vi "MoveOneStep.vi"(8 "error in (no error)":errorcluster, 11 "2D_Representer in":refnum<class "2D_Representer.lvclass">) -> (0 "error out":errorcluster, 3 "2D_Representer out":refnum<class "2D_Representer.lvclass">)   [LabVIEW 2018, in "2D_Representer.lvclass"]
uses:
  2D_Representer.lvclass
  2D_Representer.lvclass/2D_Representer.ctl
  Snake/Snake.lvclass
  Feeder/Feeder.lvclass
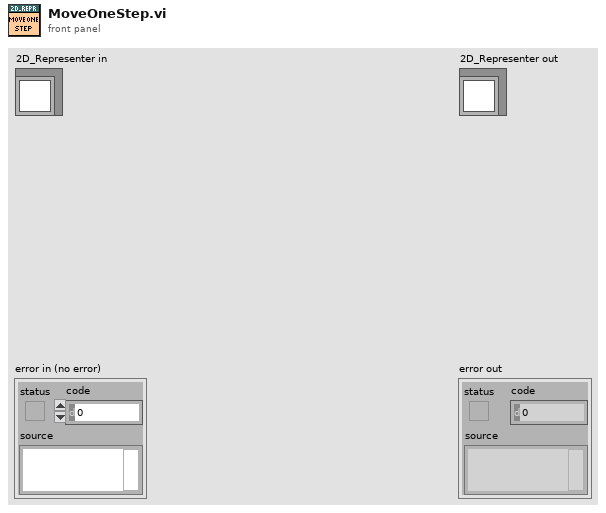
[diagram p1: front panel]
types:
  T1 = typedef "XYposition.ctl" = cluster{"Col.LocX":i32, "Row.LocY":i32}
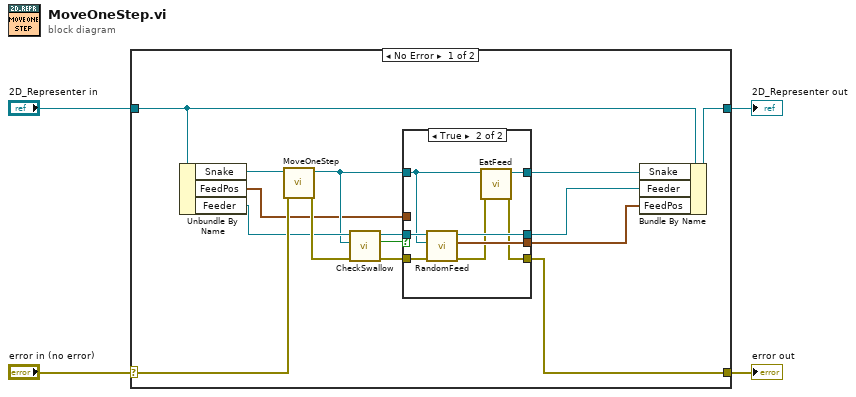
[diagram p0: block diagram]
diagram:
  n1 = case shown="No Error" "error in (no error)" {
    selector: "error in (no error)" -> [w16 w33]
    tunnel: [w12 w33] -> w3
    tunnel: [w17 w32] -> w1
    tunnel: "2D_Representer in" -> [w19 w32]
    frame No Error {
      n2 = Unbundle By Name(w19) -> ("Snake"=w18:refnum<class "Snake.lvclass">, "FeedPos"=w6:T1, "Feeder"=w13:refnum<class "Feeder.lvclass">)
      n3 = call "MoveOneStep.vi"("error in (no error)"=w16, "Snake in"=w18) -> ("error out"=w15:errorcluster, "Snake out"=w9:refnum<class "Snake.lvclass">)  [unwired: 8 in]
      n4 = call "CheckSwallow.vi"("error in (no error)"=w15, "Snake.lvclass"=w9, "Feeder in"=w13) -> ("error out"=w14:errorcluster, "Swallowed?"=w11:bool, "Feeder out"=w10:refnum<class "Feeder.lvclass">)  [unwired: 6 in]
      n5 = case shown="True" w11 {
        tunnel: w14 -> [w23 w31]
        tunnel: [w23 w24] -> w12
        tunnel: w10 -> [w22 w30]
        tunnel: w9 -> [w20 w27]
        tunnel: [w22 w29] -> w8
        tunnel: [w21 w28] -> w7
        tunnel: w6 -> [w21 _]
        tunnel: [w20 w26] -> w5
        frame False {
        }
        frame True {
          n6 = call "RandomFeed.vi"("error in (no error)"=w31, "Snake"=w27, "Feeder in"=w30) -> ("error out"=w25:errorcluster, "FeedPos"=w28:T1, "Feeder out"=w29:refnum<class "Feeder.lvclass">)  [unwired: 6 in]
          n7 = call "EatFeed.vi"("error in (no error)"=w25, "Snake in"=w27) -> ("error out"=w24:errorcluster, "Snake out"=w26:refnum<class "Snake.lvclass">)  [unwired: 8 in]
        }
      }
      n8 = Bundle By Name(cluster=w19, "Snake"=w5, "Feeder"=w8, "FeedPos"=w7) -> (w17:refnum<class "2D_Representer.lvclass">)
    }
    frame Error {
    }
  }
  "error out" <- w3
  "2D_Representer out" <- w1
